vi "Play.vi"(8 "error in (no error)":errorcluster, 11 "Data in":refnum<class "SR430Class.lvclass">) -> (0 "error out":errorcluster, 3 "Data out":refnum<class "SR430Class.lvclass">)   [LabVIEW 2015, in "SR430Class.lvclass"]
uses:
  class/SR430Class.lvclass
  class/SR430Class.lvclass/SR430Class.ctl
  support/SR430 Driver/SR430Driver.lvlib
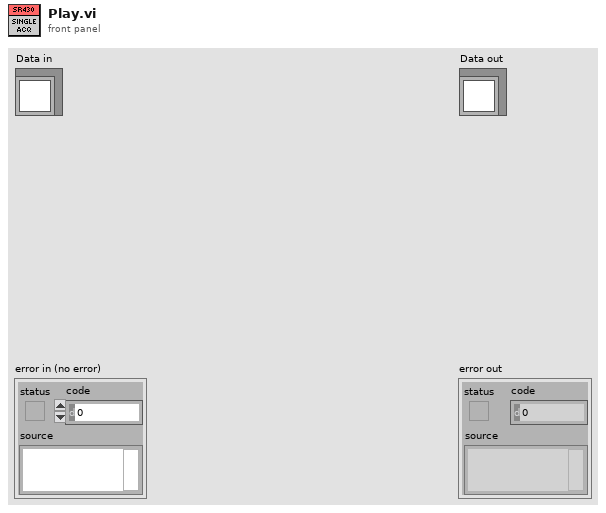
[diagram p1: front panel]
types:
  T1 = typedef "SR430Driver.lvlib/SR430_VISA Control.ctl" = cluster{"VISA resource name":refnum<visa-resource-name>}
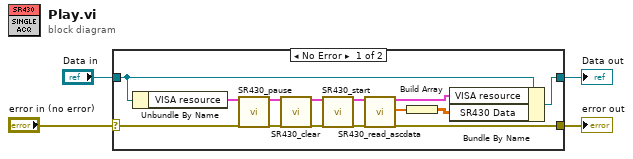
[diagram p0: block diagram]
diagram:
  n1 = case shown="No Error" "error in (no error)" {
    selector: "error in (no error)" -> [w11 w20]
    tunnel: [w10 w20] -> w3
    tunnel: [w8 w19] -> w1
    tunnel: "Data in" -> [w9 w19]
    frame No Error {
      n2 = Unbundle By Name(w9) -> ("VISA resource"=w12:T1)
      n3 = call "SR430_pause.vi"("address"=w12, "error in (no error)"=w11) -> ("address out"=w18:T1, "error out"=w17:errorcluster)  [unwired: 16 in]
      n4 = call "SR430_clear.vi"("address"=w18, "error in (no error)"=w17) -> ("address out"=w15:T1, "error out"=w16:errorcluster)  [unwired: 16 in]
      n5 = call "SR430_start.vi"("address"=w15, "error in (no error)"=w16) -> ("address out"=w14:T1, "error out"=w13:errorcluster)  [unwired: 16 in]
      n6 = call "SR430_read_ascdata.vi"("address"=w14, "error in (no error)"=w13) -> ("address out"=w5:T1, "Data"=w7:dbl[], "error out"=w10:errorcluster)  [unwired: 14 in, 1 out]
      n7 = Build Array(w7) -> (w6:dbl[][])
      n8 = Bundle By Name(cluster=w9, "VISA resource"=w5, "SR430 Data"=w6) -> (w8:refnum<class "SR430Class.lvclass">)
    }
    frame Error {
    }
  }
  "error out" <- w3
  "Data out" <- w1
